vi "FlatCase.vi"() -> ()   [LabVIEW 2020]
panel:
  in  "stop":bool
  out "led":bool
  in  "millisecond timer value":u32
  in  "milliseconds to wait":u32
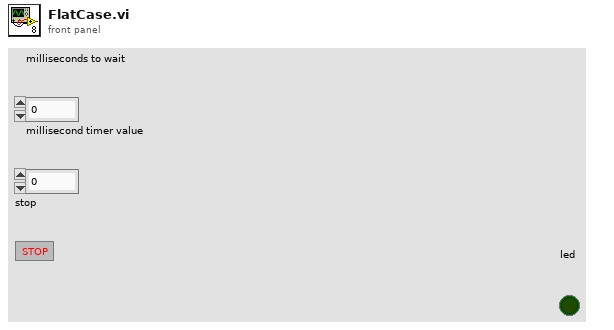
[diagram p1: front panel]
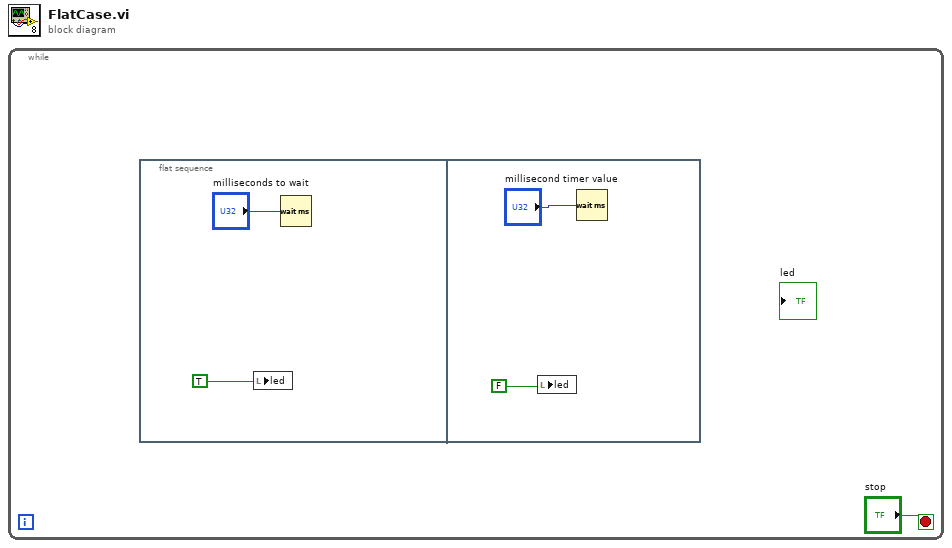
[diagram p0: block diagram]
diagram:
  n1 = while {
    stop <- "stop" stop-if-true
    n2 = flat-sequence {
      frame #0 {
        n3 = local write "led"(TRUE) -> ()
        n4 = Wait (ms)(milliseconds to wait="milliseconds to wait") -> ()  [unwired: 1 out]
      }
      frame #1 {
        n5 = local write "led"(FALSE) -> ()
        n6 = Wait (ms)(milliseconds to wait="millisecond timer value") -> ()  [unwired: 1 out]
      }
    }
  }
